vi "Wait.vi"(8 "error in":errorcluster, 10 "milliseconds to wait":u32) -> (0 "error out":errorcluster)   [LabVIEW 2013]
doc: "Waits the specified number of milliseconds. Error in/out clusters allow for flow control."
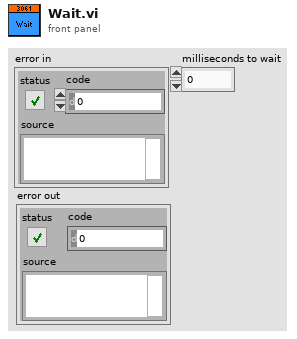
[diagram p1: front panel]
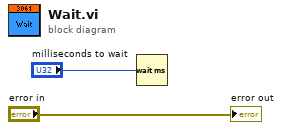
[diagram p0: block diagram]
diagram:
  n1 = Wait (ms)(milliseconds to wait="milliseconds to wait") -> ()  [unwired: 1 out]
  "error out" <- "error in"
